vi "AFT Filter Signal and Update Coefficients (Real, Array).vi"(6 "step size":dbl=-1.0, 7 "reset? (F)":bool, 8 "error in (no error)":errorcluster, 9 "d(n)":dbl[](array[numeric]), 10 "x(n)":dbl[](array[numeric]), 11 "adaptive filter in":refnum<k20>) -> (0 "error out":errorcluster, 1 "e(n)":dbl[](array[numeric]), 2 "y(n)":dbl[](array[numeric]), 3 "adaptive filter out":refnum<k20>)   [LabVIEW 2017, in "NI_AdaptiveFilter.lvlib"]
doc: "Filters an input signal with an adaptive filter and updates the coefficients of the adaptive filter iteratively. You must use the least mean squares (LMS) or recursive least squares (RLS) algorithms to create the adaptive filter. Wire data to the <B>x(n)</B> and <B>d(n)</B> inputs to determine the polymorphic instance to use or manually select the instance. The data type of the adaptive filter that you wire to the <B>adaptive filter in</B> input must match the instance of the AFT Filter Signal and Update Coefficients VI."
uses:
  <vilib>/addons/Adaptive Filters/NI_AdaptiveFilter.lvlib
  <resource>/AdaptiveFilters.dll
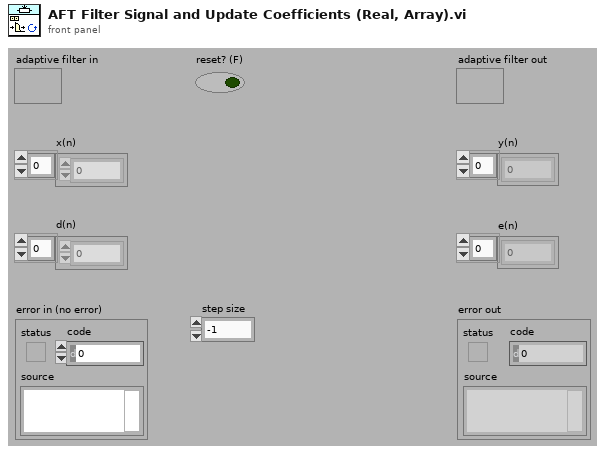
[diagram p1: front panel]
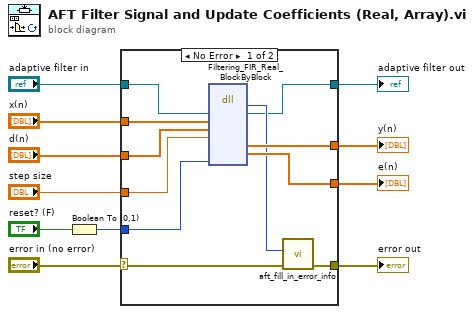
[diagram p0: block diagram]
diagram:
  n1 = Boolean To (0,1)(Boolean="reset? (F)") -> (0, 1=w9:i16)
  n2 = case shown="No Error" "error in (no error)" {
    selector: "error in (no error)" -> [w18 w24]
    tunnel: [w16 w24] -> w11
    tunnel: "adaptive filter in" -> [w13 w23]
    tunnel: "x(n)" -> [w22 _]
    tunnel: "d(n)" -> [w21 _]
    tunnel: [w20 _] -> w2
    tunnel: [w19 _] -> w1
    tunnel: [w12 w23] -> w6
    tunnel: w9 -> [w15 _]
    tunnel: "step size" -> [w14 _]
    frame No Error {
      n3 = dll-call lib="C:/Program Files/National Instruments/LabVIEW 2017/resource/AdaptiveFilters.dll" fn="Filtering_FIR_Real_BlockByBlock"("pSession"=w13, "x"=w22, "d"=w21, "mu"=w14, "reset"=w15) -> ("err"=w17:i32, "pSession"=w12:refnum<k20>, "y"=w20:dbl[], "e"=w19:dbl[])  [unwired: 7 in, 4 out]
      n4 = call <vilib>:"aft_fill_in_error_info.vi"("error in"=w18, "status code"=w17) -> ("error out"=w16:errorcluster)  [unwired: 2 in, 7 out]
    }
    frame Error {
    }
  }
  "error out" <- w11
  "adaptive filter out" <- w6
  "y(n)" <- w2
  "e(n)" <- w1
